vi "String_to_num (SubVI).vi"(0 "String in":string, 2 "error in":errorcluster) -> (6 "Rest of string OUT":string, 7 "error out":errorcluster, 9 "output cluster \nof coefficients":T1 {"k1" format="%#_16g"; "k2" format="%#_16g"; "k3" format="%#_16g"; "k4" format="%#_16g"; "k5" format="%#_16g"; "k6" format="%#_16g"; "k7" format="%#_16g"; "R" format="%#_16g"})   [LabVIEW 2013]
panel:
  out "k4":dbl
  out "R":dbl
  out "k7":dbl
  out "k6":dbl
  out "k5":dbl
  out "k3":dbl
  out "k2":dbl
  out "k1":dbl
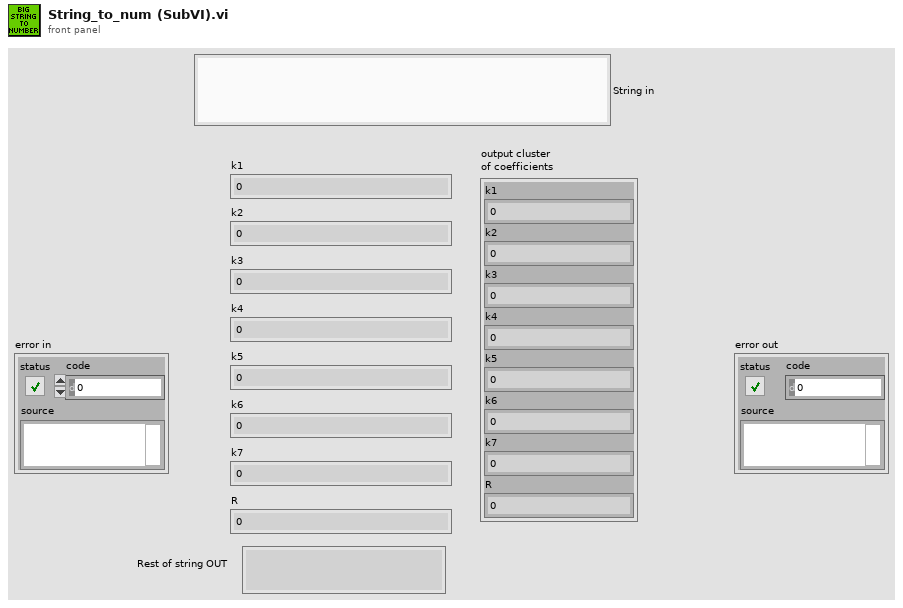
[diagram p1: front panel]
types:
  T1 = cluster{"k1":dbl, "k2":dbl, "k3":dbl, "k4":dbl, "k5":dbl, "k6":dbl, "k7":dbl, "R":dbl}
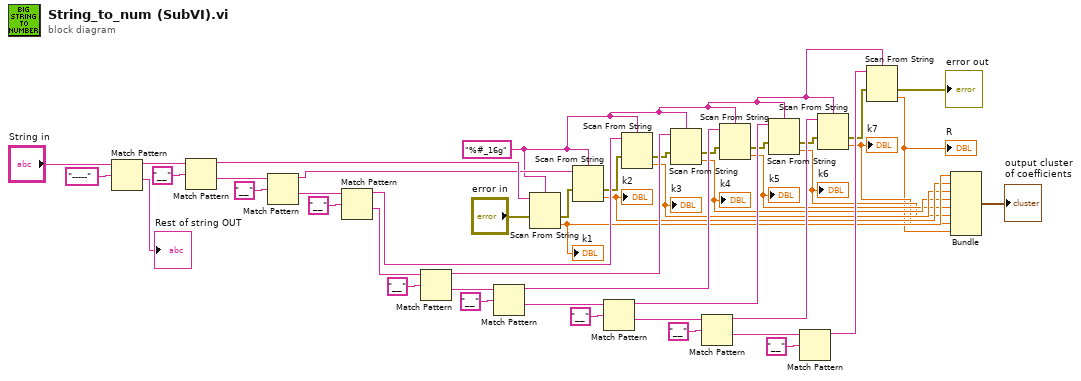
[diagram p0: block diagram]
diagram:
  w12 = "%#_16g" ("format string")
  n1 = Match Pattern(string="String in", regular expression="-----") -> (before substring=w31:string, after substring=→"Rest of string OUT":string)  [unwired: 1 in, 2 out]
  n2 = Match Pattern(string=w31, regular expression="__" ("delimiter (Tab)")) -> (before substring=w27:string, after substring=w39:string)  [unwired: 1 in, 2 out]
  n3 = Match Pattern(string=w39, regular expression="__" ("delimiter (Tab)")) -> (before substring=w26:string, after substring=w32:string)  [unwired: 1 in, 2 out]
  n4 = Match Pattern(string=w32, regular expression="__" ("delimiter (Tab)")) -> (before substring=w25:string, after substring=w33:string)  [unwired: 1 in, 2 out]
  n5 = Match Pattern(string=w33, regular expression="__" ("delimiter (Tab)")) -> (before substring=w24:string, after substring=w34:string)  [unwired: 1 in, 2 out]
  n6 = Match Pattern(string=w34, regular expression="__" ("delimiter (Tab)")) -> (before substring=w23:string, after substring=w35:string)  [unwired: 1 in, 2 out]
  n7 = Scan From String(format string=w12, input string=w27, error in="error in") -> (error out=w19:errorcluster, output 1=w9:dbl)  [unwired: 2 in, 2 out]
  "k1" <- w9
  n8 = Scan From String(format string=w12, input string=w26, error in=w19) -> (error out=w18:errorcluster, output 1=w8:dbl)  [unwired: 2 in, 2 out]
  "k2" <- w8
  n9 = Match Pattern(string=w35, regular expression="__" ("delimiter (Tab)")) -> (before substring=w22:string, after substring=w36:string)  [unwired: 1 in, 2 out]
  n10 = Scan From String(format string=w12, input string=w25, error in=w18) -> (error out=w17:errorcluster, output 1=w7:dbl)  [unwired: 2 in, 2 out]
  "k3" <- w7
  n11 = Scan From String(format string=w12, input string=w24, error in=w17) -> (error out=w16:errorcluster, output 1=w6:dbl)  [unwired: 2 in, 2 out]
  "k4" <- w6
  n12 = Match Pattern(string=w36, regular expression="__" ("delimiter (Tab)")) -> (before substring=w21:string, after substring=w37:string)  [unwired: 1 in, 2 out]
  n13 = Scan From String(format string=w12, input string=w23, error in=w16) -> (error out=w15:errorcluster, output 1=w5:dbl)  [unwired: 2 in, 2 out]
  "k5" <- w5
  n14 = Scan From String(format string=w12, input string=w22, error in=w15) -> (error out=w14:errorcluster, output 1=w4:dbl)  [unwired: 2 in, 2 out]
  "k6" <- w4
  n15 = Match Pattern(string=w37, regular expression="__" ("delimiter (Tab)")) -> (before substring=w20:string)  [unwired: 1 in, 3 out]
  n16 = Scan From String(format string=w12, input string=w21, error in=w14) -> (error out=w13:errorcluster, output 1=w3:dbl)  [unwired: 2 in, 2 out]
  "k7" <- w3
  n17 = Scan From String(format string=w12, input string=w20, error in=w13) -> (error out=→"error out":errorcluster, output 1=w2:dbl)  [unwired: 2 in, 2 out]
  "R" <- w2
  n18 = Bundle("k1"=w9, "k2"=w8, "k3"=w7, "k4"=w6, "k5"=w5, "k6"=w4, "k7"=w3, "R"=w2) -> (→"output cluster \nof coefficients":T1)  [unwired: 1 in]
